vi "SRingStartFetch.vi"   [LabVIEW 2015]
uses:
  ESLSCDLL.dll
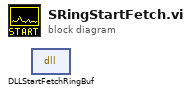
[diagram p0: block diagram]
diagram:
  n1 = dll-call lib="C:/ENTW/PCIE/64bit/lv64/1cam/board.vis/ESLSCDLL.dll" fn="DLLStartFetchRingBuf"() -> ()  [unwired: 4 in, 2 out]
